vi "set_settings_cluster.vi"(8 "error in (no error)":errorcluster, 10 "settings cluster variant":variant, 11 "DataCollectionDL110128Streaming in":refnum<class "DataCollectionDL110128Streaming.lvclass">) -> (0 "error out":errorcluster, 3 "DataCollectionDL110128Streaming out":refnum<class "DataCollectionDL110128Streaming.lvclass">)   [LabVIEW 2010, in "DataCollectionDL110128Streaming.lvclass"]
uses:
  DataCollectionDL110128Streaming.lvclass
  DataCollectionDL110128Streaming.lvclass/DataCollectionDL110128Streaming.ctl
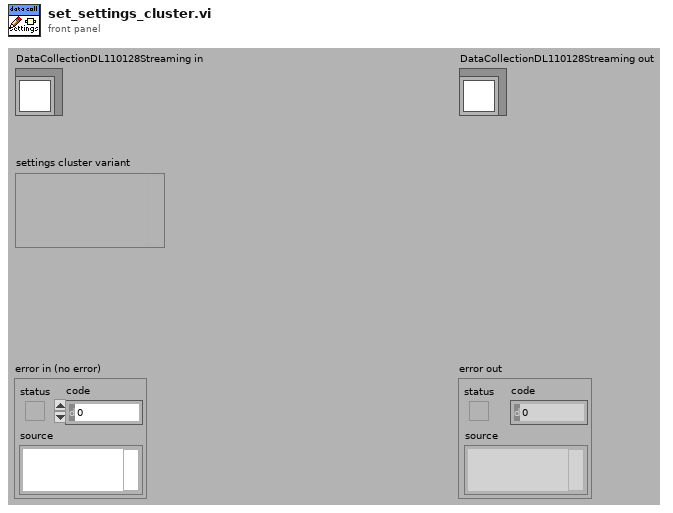
[diagram p1: front panel]
types:
  T1 = typedef "DataCollectionDL110128Streaming.lvclass/settings_cluster.ctl" = cluster{"autosave?":bool}
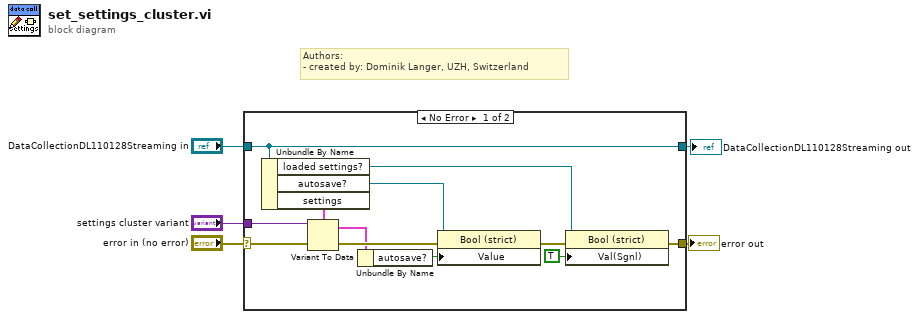
[diagram p0: block diagram]
diagram:
  # "Authors: \n- created by: Dominik Langer, UZH, Switzerland"
  n1 = case shown="No Error" "error in (no error)" {
    selector: "error in (no error)" -> [w17 w18]
    tunnel: "DataCollectionDL110128Streaming in" -> [w10 w19]
    tunnel: "settings cluster variant" -> [w16 _]
    tunnel: [w11 w18] -> w2
    tunnel: [w10 w19] -> w1
    frame No Error {
      n2 = Unbundle By Name(w10) -> ("loaded settings?"=w9:refnum<vi>, "autosave?"=w8:refnum<vi>, "settings"=w15:T1)
      n3 = Variant To Data(error in=w17, Variant=w16, type=w15) -> (error out=w14:errorcluster, data=w13:T1)
      n4 = Unbundle By Name(w13) -> ("autosave?"=w7:bool)
      n5 = property class="Bool (strict)"(reference=w8, error in=w14, "Value"=w7) -> (error out=w12:errorcluster)  [unwired: 1 out]
      n6 = property class="Bool (strict)"(reference=w9, error in=w12, "Val(Sgnl)"=TRUE) -> (error out=w11:errorcluster)  [unwired: 1 out]
    }
    frame Error {
    }
  }
  "error out" <- w2
  "DataCollectionDL110128Streaming out" <- w1
